vi "SetMeasureAutozero.vi"(7 "SMU":T1, 8 "Error In":errorcluster, 10 "Autozero Mode":T2, 11 "Keithley 2602 In":refnum<visa-resource-name>) -> (0 "Error Out":errorcluster, 3 "Keithley 2602 Out":refnum<visa-resource-name>)   [LabVIEW 2012, in "Keithley-2602.lvlib"]
uses:
  Keithley-2602.lvlib
  Controls/AutozeroMode.ctl
  Controls/SMU.ctl
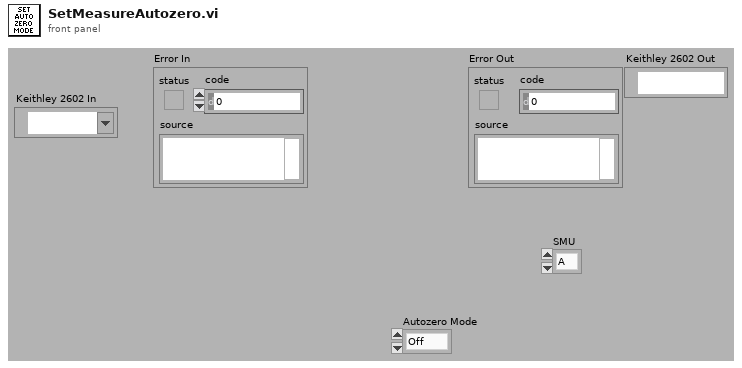
[diagram p1: front panel]
types:
  T1 = typedef "Keithley-2602.lvlib/SMU.ctl" = enum16{"A", "B"}
  T2 = typedef "Keithley-2602.lvlib/AutozeroMode.ctl" = enum16{"Off", "Once", "Auto"}
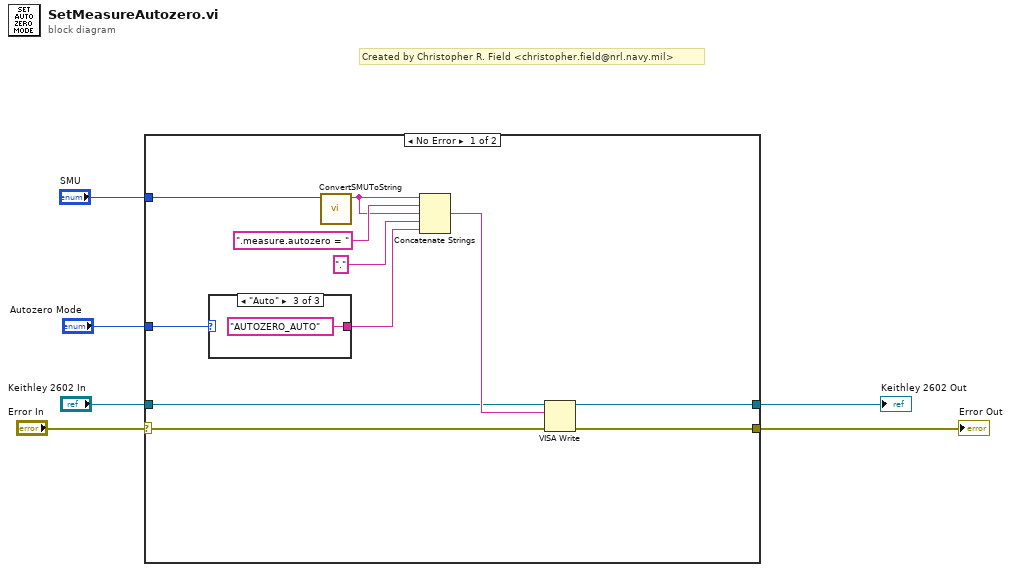
[diagram p0: block diagram]
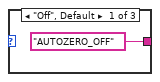
[diagram p2: hidden frame]
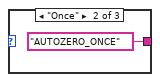
[diagram p3: hidden frame]
diagram:
  # "Created by Christopher R. Field <christopher.field@nrl.navy.mil>"
  n1 = case shown="No Error" "Error In" {
    selector: "Error In" -> [w7 w21]
    tunnel: "Keithley 2602 In" -> [w15 w22]
    tunnel: [w14 w21] -> w5
    tunnel: [w13 w22] -> w4
    tunnel: "SMU" -> [w9 _]
    tunnel: "Autozero Mode" -> [w8 _]
    frame No Error {
      n2 = case shown="\"Auto\"" w8 {
        tunnel: ["AUTOZERO_OFF" "AUTOZERO_ONCE" "AUTOZERO_AUTO"] -> w10
        frame "Off", Default {
        }
        frame "Once" {
        }
        frame "Auto" {
        }
      }
      n3 = call "ConvertSMUToString.vi"("SMU"=w9) -> ("Channel"=w12:string)  [unwired: 10 in]
      n4 = Concatenate Strings(w12, ".measure.autozero = ", w12, "." ("string"), w10) -> (w16:string)
      n5 = VISA Write(VISA resource name=w15, write buffer=w16, error in (no error)=w7) -> (VISA resource name out=w13:refnum<visa-resource-name>, error out=w14:errorcluster)  [unwired: 1 out]
    }
    frame Error {
    }
  }
  "Error Out" <- w5
  "Keithley 2602 Out" <- w4
